vi "Robo Wait for Stream Command ended.vi"(7 "Timeout":u32=30000, 10 "Command":string, 11 "Notifier in":refnum<notifier>) -> (0 "error out":errorcluster)   [LabVIEW 2015]
uses:
  Robo Team Engine Command.ctl
  Robo Team Globals.vi
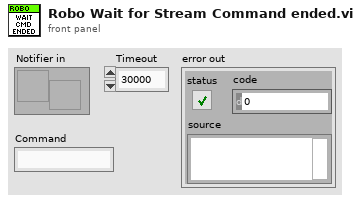
[diagram p1: front panel]
types:
  T1 = typedef "Robo Team Engine Command.ctl" = cluster{"Command":string, "Data":variant, "Error":errorcluster, "Timeout":i32}
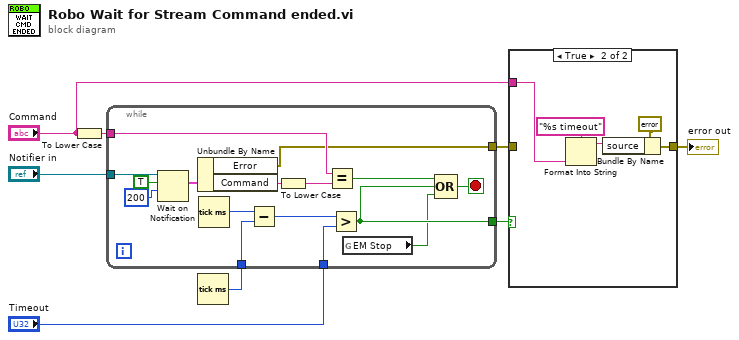
[diagram p0: block diagram]
diagram:
  n1 = To Lower Case(string="Command") -> (all lower case string=w1:string)
  n2 = Tick Count (ms)() -> (millisecond timer value=w7:u32)
  n3 = while {
    tunnel: "Notifier in" -> [w24]
    tunnel: w1 -> [w20]
    tunnel: w7 -> [w17]
    tunnel: [w13] -> w4
    tunnel: "Timeout" -> [w12]
    tunnel: [w11] -> w5
    stop <- w14 stop-if-true
    n4 = Wait on Notification(notifier=w24, ignore previous (F)=TRUE, timeout in ms (-1)=200) -> (notification=w22:T1)  [unwired: 1 in, 3 out]
    n5 = Unbundle By Name(w22) -> ("Error"=w13:errorcluster, "Command"=w21:string)
    n6 = Tick Count (ms)() -> (millisecond timer value=w18:u32)
    n7 = Subtract(x=w18, y=w17) -> (x-y=w16:u32)
    n8 = To Lower Case(string=w21) -> (all lower case string=w9:string)
    n9 = Equal?(x=w20, y=w9) -> (x = y?=w15:bool)
    n10 = Greater?(x=w16, y=w12) -> (0:w11:bool)
    n11 = global read "Robo Team Globals.vi" "EM Stop"() -> (w10:bool)
    n12 = Compound Arithmetic op=OR(w15, w11, w10) -> (w14:bool)
  }
  n13 = case shown="True" w5 {
    tunnel: w4 -> [w25 _]
    tunnel: [w25 w28] -> w3
    tunnel: "Command" -> [_ w30]
    frame False {
    }
    frame True {
      n14 = Format Into String(format string="%s timeout", w30) -> (resulting string=w26:string)  [unwired: 2 in, 1 out]
      n15 = Bundle By Name(cluster=errorcluster {"status"=TRUE, "code"=7001, "source"="Timeout"} ("Error"), "source"=w26) -> (w28:errorcluster)
    }
  }
  "error out" <- w3
